vi "Self-Test.vi"(8 "error in (no error)":errorcluster, 11 "VISA resource name":refnum<visa-resource-name>) -> (0 "error out":errorcluster, 3 "VISA resource name out":refnum<visa-resource-name>)   [LabVIEW 2020, in "3458A Basic Driver.lvlib"]
doc: "Runs the instrument's self-test routine. If there was an error, the error out indicator shows the error code and string and the front panel displays \"Self Test Failed\". If there was no error, then the front panel displays the string \"Self Test Passed\"."
uses:
  3458A Basic Driver.lvlib
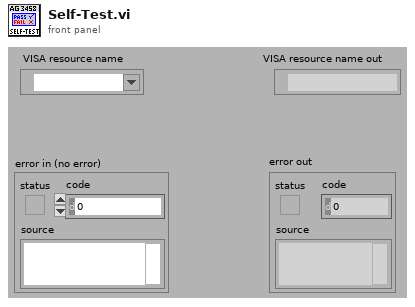
[diagram p1: front panel]
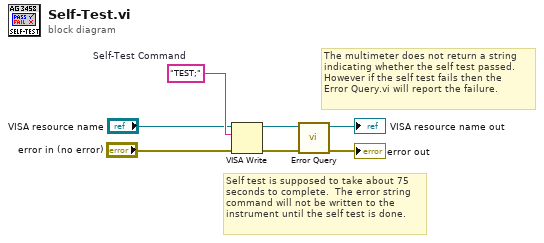
[diagram p0: block diagram]
diagram:
  w6 = "TEST;"  # Self-Test Command
  # "The multimeter does not return a string \nindicating whether the self test passed.\nHowever if the self test fails then the\nError Query.vi will report the failure."
  # "Self test is supposed to take about 75\nseconds to complete.  The error string\ncommand will not be written to the \ninstrument until the self test is done."
  n1 = VISA Write(VISA resource name="VISA resource name", write buffer=w6, error in (no error)="error in (no error)") -> (VISA resource name out=w4:refnum<visa-resource-name>, error out=w3:errorcluster)  [unwired: 1 out]
  n2 = call "Error Query.vi"("error in (no error)"=w3, "VISA resource name"=w4) -> ("error out"=→"error out":errorcluster, "VISA resource name out"=→"VISA resource name out":refnum<visa-resource-name>)  [unwired: 6 in, 2 out]
